vi "OpenWebSocketCommunication.vi"(5 "timeout hand shake [ms]":i32=5000, 6 "wait for reply (T)":bool=TRUE, 7 "timeout opening [ms]":i32=5000, 8 "error in":errorcluster, 9 "WS Server Port":string="25010", 10 "WS Server IP":string="ws://127.0.0.1") -> (0 "error out":errorcluster, 1 "timed out?":bool, 3 "Return Headers":variant)   [LabVIEW 2023, in "DeviceManager.lvlib"]
doc: "This event opens the websocket communcation from the DeviceManager to the ICL.exe\n_____\nCreated using DQMH Event Scripter 7.0.0.1280."
uses:
  DeviceManager.lvlib
  OpenWebSocketCommunication Argument--cluster.ctl
  OpenWebSocketCommunication (Reply Payload)--cluster.ctl
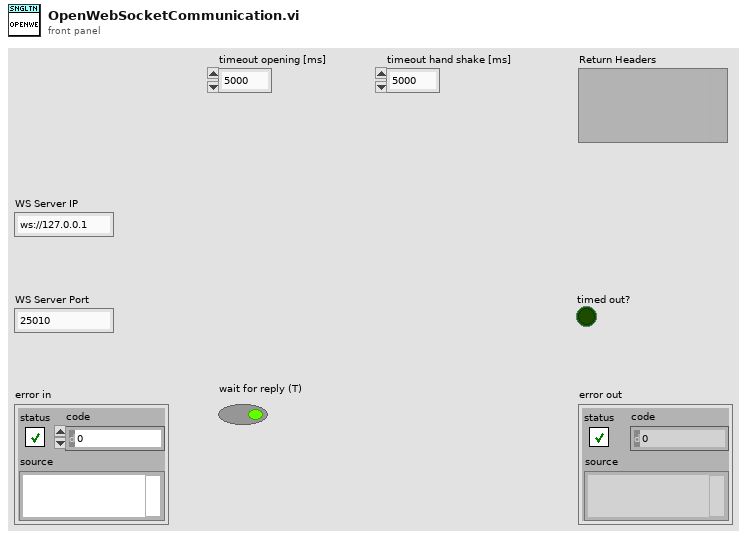
[diagram p1: front panel]
types:
  T1 = typedef "DeviceManager.lvlib/OpenWebSocketCommunication Argument--cluster.ctl" = cluster{"WS Server IP":string, "WS Server Port":string, "timeout opening [ms]":i32, "timeout hand shake [ms]":i32, "Wait Notifier":refnum<notifier>, "wait for reply":bool}
  T2 = typedef "DeviceManager.lvlib/Request Events--cluster.ctl" = cluster{"Stop Module":refnum<user-event>, "Show Panel":refnum<user-event>, "Hide Panel":refnum<user-event>, "Get Module Execution Status":refnum<user-event>, "Show Diagram":refnum<user-event>, "StartICL":refnum<user-event>, "OpenWebSocketCommunication":refnum<user-event>}
  T3 = typedef "DeviceManager.lvlib/OpenWebSocketCommunication (Reply Payload)--cluster.ctl" = cluster{"Return Headers":variant, "error":errorcluster}
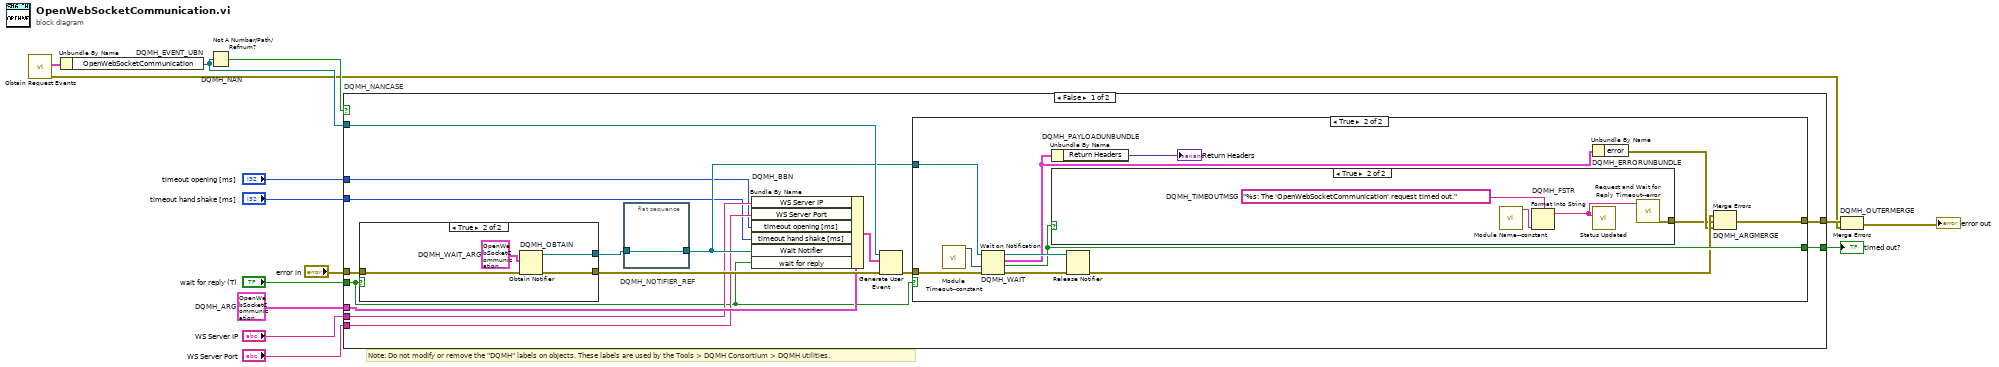
[diagram p0: block diagram]
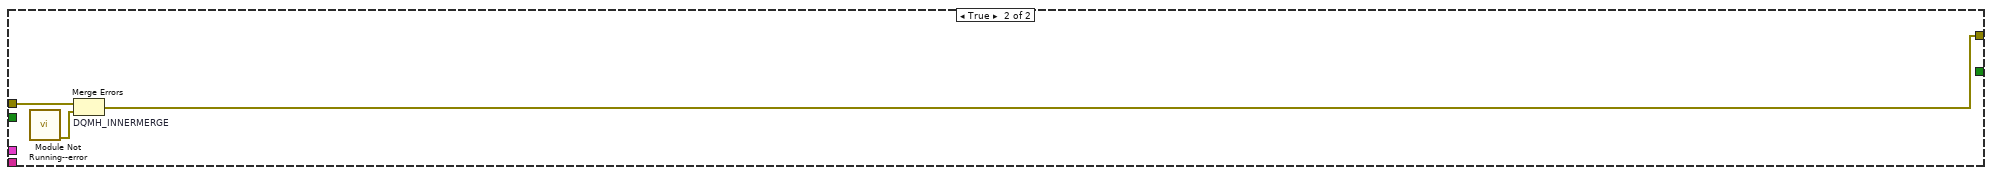
[diagram p5: hidden frame]
diagram:
  w8 = T1 {"WS Server IP"="ws://127.0.0.1", "WS Server Port"="25010", "timeout opening [ms]"=5000, "timeout hand shake [ms]"=5000, "Wait Notifier"=refnum, "wait for reply"=FALSE}  # DQMH_ARG
  # "Note: Do not modify or remove the \"DQMH\" labels on objects. These labels are used by the Tools > DQMH Consortium > DQMH utilities."
  n1 = call "Obtain Request Events.vi"() -> ("error out"=w2:errorcluster, "DeviceManager Request Events"=w1:T2)  [unwired: 10 in]
  n2 = Unbundle By Name "DQMH_EVENT_UBN"(w1) -> ("OpenWebSocketCommunication"=w12:refnum<user-event>)
  n3 = Not A Number/Path/Refnum? "DQMH_NAN"(number/path/refnum=w12) -> (NaN/Path/Refnum?=w11:bool)
  n4 = case "DQMH_NANCASE" shown="False" w11 {
    tunnel: "error in" -> [w29 w55]
    tunnel: w12 -> [w27 _]
    tunnel: [w24 w54] -> w9
    tunnel: [w25 _] -> w10
    tunnel: w8 -> [w20 _]
    tunnel: "WS Server IP" -> [w19 _]
    tunnel: "WS Server Port" -> [w18 _]
    tunnel: "timeout opening [ms]" -> [w17 _]
    tunnel: "timeout hand shake [ms]" -> [w16 _]
    tunnel: "wait for reply (T)" -> [w15 _]
    frame False {
      n5 = case shown="True" w15 {
        tunnel: w29 -> [w48 w52]
        tunnel: [w48 w51] -> w26
        tunnel: [_ w49] -> w22
        frame False {
        }
        frame True {
          w50 = T3 {"Return Headers"=variant, "error"={"status"=FALSE, "code"=0, "source"=""}}  # DQMH_WAIT_ARG
          n6 = Obtain Notifier "DQMH_OBTAIN"(notification data type=w50, error in (no error)=w52) -> (notifier out=w49:refnum<notifier>, error out=w51:errorcluster)  [unwired: 2 in, 1 out]
        }
      }
      n7 = flat-sequence "DQMH_NOTIFIER_REF" {
        tunnel: w22 -> [w30]
        tunnel: [w30] -> w21
        frame #0 {
        }
      }
      n8 = Bundle By Name "DQMH_BBN"(cluster=w20, "WS Server IP"=w19, "WS Server Port"=w18, "timeout opening [ms]"=w17, "timeout hand shake [ms]"=w16, "Wait Notifier"=w21, "wait for reply"=w15) -> (w23:T1)
      n9 = Generate User Event(user event=w27, event data cluster=w23, error in=w26) -> (error out=w28:errorcluster)  [unwired: 1 in, 1 out]
      n10 = case shown="True" w15 {
        tunnel: w28 -> [w31 w43]
        tunnel: w21 -> [_ w42]
        tunnel: [_ w40] -> w25
        tunnel: [w31 w39] -> w24
        frame False {
        }
        frame True {
          n11 = call "Module Timeout--constant.vi"() -> ("Module Timeout"=w33:i32)  [unwired: 11 in]
          n12 = Wait on Notification "DQMH_WAIT"(notifier=w42, timeout in ms (-1)=w33, error in (no error)=w43) -> (notifier out=w41:refnum<notifier>, notification=w34:T3, timed out?=w40:bool, error out=w38:errorcluster)  [unwired: 1 in]
          n13 = Unbundle By Name "DQMH_PAYLOADUNBUNDLE"(w34) -> ("Return Headers"=→"Return Headers":variant)
          n14 = case shown="True" w40 {
            tunnel: [_ w45] -> w35
            frame False {
            }
            frame True {
              w47 = "%s: The 'OpenWebSocketCommunication' request timed out."  # DQMH_TIMEOUTMSG
              n15 = call "Module Name--constant.vi"() -> ("Module Name"=w44:string)  [unwired: 11 in]
              n16 = Format Into String "DQMH_FSTR"(format string=w47, w44) -> (resulting string=w46:string)  [unwired: 2 in, 1 out]
              n17 = call "Status Updated.vi"("Status"=w46) -> ()  [unwired: 10 in, 1 out]
              n18 = call "Request and Wait for Reply Timeout--error.vi"("Error Message"=w46) -> ("error out"=w45:errorcluster)  [unwired: 10 in]
            }
          }
          n19 = Release Notifier(notifier=w41, error in (no error)=w38) -> (error out=w37:errorcluster)  [unwired: 1 in, 2 out]
          n20 = Unbundle By Name "DQMH_ERRORUNBUNDLE"(w34) -> ("error"=w36:errorcluster)
          n21 = Merge Errors "DQMH_ARGMERGE"(w37, w35, w36) -> (w39:errorcluster)
        }
      }
    }
    frame True {
      n22 = call "Module Not Running--error.vi"() -> ("error out"=w53:errorcluster)  [unwired: 11 in]
      n23 = Merge Errors "DQMH_INNERMERGE"(w55, w53) -> (w54:errorcluster)
    }
  }
  "timed out?" <- w10
  n24 = Merge Errors "DQMH_OUTERMERGE"(w9, w2) -> (→"error out":errorcluster)
